vi "Set Exclusions.vi"(4 "Exclude dependent shared libraries":bool, 6 "Exclude dependent packed libraries":bool, 8 "error in (no error)":errorcluster, 9 "Disconnect inline subVIs":bool, 10 "Exclusions":T1, 11 "SDIST in":refnum<class "NI_AB_API_DSDIST.lvclass">) -> (0 "error out":errorcluster, 3 "SDIST out":refnum<class "NI_AB_API_DSDIST.lvclass">)   [LabVIEW 2020, in "NI_AB_API_DSDIST.lvclass"]
uses:
  <vilib>/AppBuilder/AB_API/DSDIST/NI_AB_API_DSDIST.lvclass
  <vilib>/AppBuilder/AB_API/common/AB_API Primary Exclusions.ctl
  <vilib>/AppBuilder/AB_API/SDIST/NI_AB_API_SDIST.lvclass
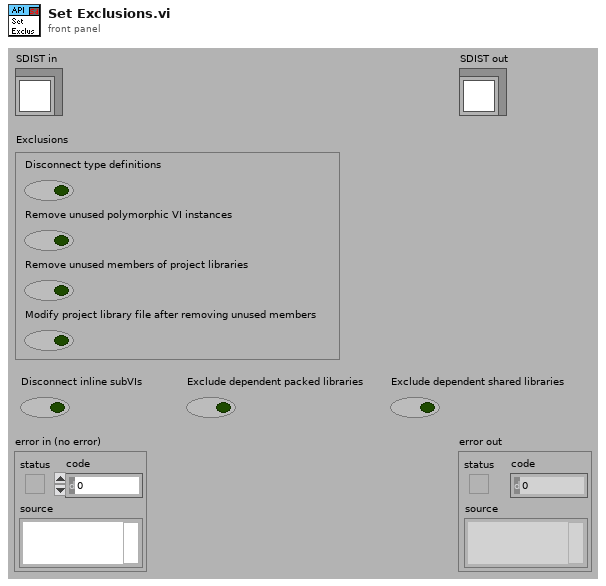
[diagram p1: front panel]
types:
  T1 = typedef "AB_API Primary Exclusions.ctl" = cluster{"Disconnect type definitions":bool, "Remove unused polymorphic VI instances":bool, "Remove unused members of project libraries":bool, "Modify project library file after removing unused members":bool}
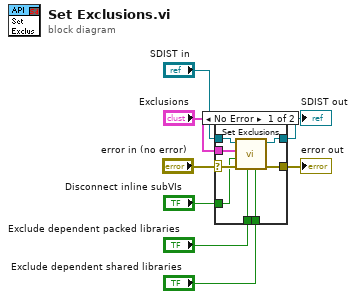
[diagram p0: block diagram]
diagram:
  n1 = case shown="No Error" "error in (no error)" {
    selector: "error in (no error)" -> [w14 w18]
    tunnel: [w13 w18] -> w7
    tunnel: [w15 w17] -> w5
    tunnel: "SDIST in" -> [w16 w17]
    tunnel: "Exclusions" -> [w12 _]
    tunnel: "Disconnect inline subVIs" -> [w11 _]
    tunnel: "Exclude dependent packed libraries" -> [w10 _]
    tunnel: "Exclude dependent shared libraries" -> [w9 _]
    frame No Error {
      n2 = call-parent "Set Exclusions.vi"("Exclude dependent shared libraries"=w9, "Exclude dependent packed libraries"=w10, "error in (no error)"=w14, "Disconnect inline subVIs"=w11, "Exclusions"=w12, "SDIST in"=w16) -> ("error out"=w13:errorcluster, "SDIST out"=w15:refnum<class "NI_AB_API_DSDIST.lvclass">)  [unwired: 4 in]
    }
    frame Error {
    }
  }
  "error out" <- w7
  "SDIST out" <- w5
